vi "VisionMode.vi"(2 "ModeIn":string) -> (0 "ModeOut":string)   [LabVIEW 2016]
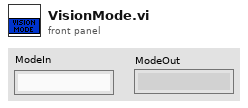
[diagram p1: front panel]
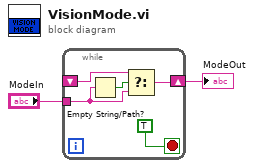
[diagram p0: block diagram]
diagram:
  n1 = while {
    shift-right: [w5] -> w2
    shift-left: _ -> [w6]
    tunnel: "ModeIn" -> [w3]
    stop <- TRUE stop-if-true
    n2 = Empty String/Path?(string/path=w3) -> (empty?=w4:bool)
    n3 = Select(t=w6, s=w4, f=w3) -> (s? t:f=w5:string)
  }
  "ModeOut" <- w2
